vi "SLSC_InitSession.vi"() -> ()   [LabVIEW 2021]
uses:
  <vilib>/httpClient/POSTBuffer.vi
  <vilib>/httpClient/LabVIEWHTTPClient.lvlib
panel:
  out "error out":errorcluster
  out "headers":string
  out "body":string
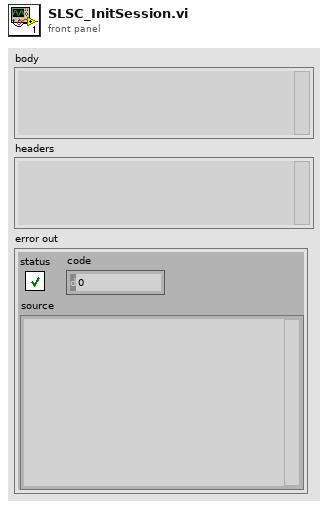
[diagram p1: front panel]
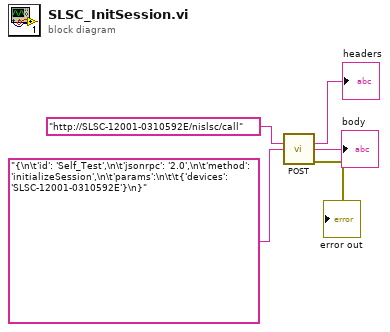
[diagram p0: block diagram]
diagram:
  n1 = call-poly <vilib>:"POST.vi"("url"="http://SLSC-12001-0310592E/nislsc/call", "buffer"="{\n\t'id': 'Self_Test',\n\t'jsonrpc': '2.0',\n\t'method': 'initializeSession',\n\t'params':\n\t\t{'devices': 'SLSC-12001-0310592E'}\n}" ("url")) -> ("headers"=→"headers":string, "body"=→"body":string, "error out"=→"error out":errorcluster)  [unwired: 10 in, 1 out]
